vi "CaLabDisconnect_PV.vi"(10 "All PVs? (No)":bool, 11 "PV Name":string) -> ()   [LabVIEW 2020, in "CaLab.lvlib"]
doc: "This is a VI for disconnecting EPICS variables.\n\n<b>INPUT:</b>\n <b>PV Name(s)</b>\n String array of EPICS variable names\n <b>all (false)</b>\n TRUE: Disconnect all EPICS variables"
uses:
  CaLab.lvlib
  calab.dll
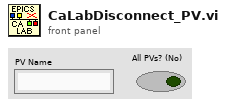
[diagram p1: front panel]
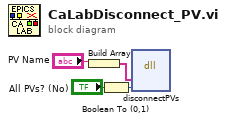
[diagram p0: block diagram]
diagram:
  n1 = Build Array("PV Name") -> (w1:string[])
  n2 = Boolean To (0,1)(Boolean="All PVs? (No)") -> (0, 1=w3:i16)
  n3 = dll-call lib="calab.dll" fn="disconnectPVs" label="caLabDisconnect"("PVNameArray"=w1, "All"=w3) -> ()  [unwired: 5 in, 3 out]
